vi "FBCF.vi"(9 "N":i32=100 min=0, 10 "g":dbl=0.7 min=0.0 max=0.95, 11 "Data in":dbl[](array[numeric]) format="%#_13g") -> (3 "Data out":dbl[](array[numeric]) format="%#_13g")   [LabVIEW 2025]
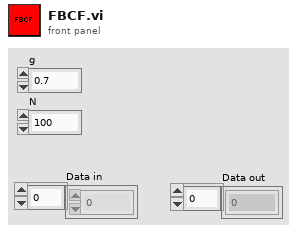
[diagram p1: front panel]
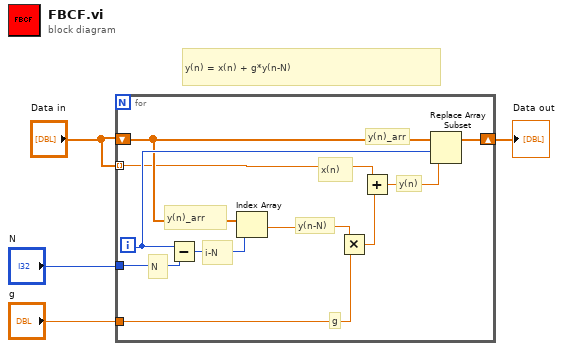
[diagram p0: block diagram]
diagram:
  # "y(n) = x(n) + g*y(n-N)"
  n1 = for {
    shift-right: [w14] -> w1
    shift-left: "Data in" -> [w6]
    tunnel: "N" -> [w9]
    tunnel: "g" -> [w7]
    tunnel: "Data in" -> [w5] mode=indexing
    i -> [w12]
    # "x(n)"
    # "i-N"
    # "y(n)_arr"
    # "N"
    # "y(n)"
    # "y(n)_arr"
    # "y(n-N)"
    # "g"
    n2 = Subtract(x=w12, y=w9) -> (x-y=w10:i32)
    n3 = Index Array(array=w6, index=w10) -> (element=w11:dbl)
    n4 = Multiply(x=w11, y=w7) -> (x*y=w8:dbl)
    n5 = Add(x=w5, y=w8) -> (x+y=w13:dbl)
    n6 = Replace Array Subset(array=w6, new element=w13, index=w12) -> (w14:dbl[])
  }
  "Data out" <- w1
